vi "SWERVE_DRIVE_GET_MAX.vi"() -> (1 "Max Rotational Vel (Rad/Sec)":dbl=1.0, 3 "Max Wheel Vel (Meter/Sec)":dbl=1.0)   [LabVIEW 2020]
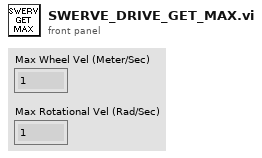
[diagram p1: front panel]
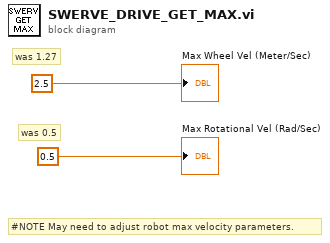
[diagram p0: block diagram]
diagram:
  # "#NOTE May need to adjust robot max velocity parameters."
  # "was 0.5"
  # "was 1.27"
  "Max Wheel Vel (Meter/Sec)" <- 2.5
  "Max Rotational Vel (Rad/Sec)" <- 0.5
